vi "PH_IEEE1394Camera.PC Show Image.vi"(0 "i ref in":refnum<vi>, 2 "Show Image":bool, 5 "error IO":errorcluster) -> (14 "i ref out":refnum<vi>, 19 "error out":errorcluster)   [LabVIEW 2014]
doc: "This is the Proc Case \"Show Image\"."
uses:
  PH_IEEE1394Camera.lvlib
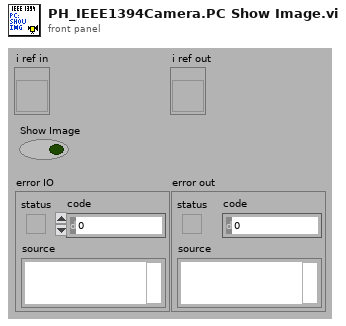
[diagram p1: front panel]
types:
  T1 = typedef "PH_IEEE1394Camera.lvlib/PH_IEEE1394Camera.i attribute.ctl" = cluster{"Gui Refs":cluster{"Cam name (Machinery)":refnum<vi>, "Start Cam":refnum<vi>, "Brightness":refnum<vi>, "Shutter":refnum<vi>, "Gain":refnum<vi>, "Center of Gravity":refnum<vi>, "Serial No":refnum<vi>, "Cam Name":refnum<vi>, "Connect":refnum<vi>, "Cam Attributes":refnum<vi>, "Supported Video Modes":refnum<vi>, "Cam Model":refnum<vi>, "Trigger Polarity":refnum<vi>, "Trigger Mode":refnum<vi>, "Trigger Timeout":refnum<vi>, "Bit Depth":refnum<vi>, "Video Mode":refnum<vi>, "Top":refnum<vi>, "Bottom":refnum<vi>, "Left":refnum<vi>, "Right":refnum<vi>, "Set ROI to Maximum":refnum<vi>}, "Cam":cluster{"Name (machinery)":string, "Serial Number":dbl, "IMAQ1394 Session":T2, "Restart":bool, "Supported Video Modes":cluster{"Video Mode":u32, "Video Mode Name":string}[], "Cam Model":string, "Readable Attributes":cluster{"Attribute Type":T3, "Attribute Name":string}[], "Writable Attributes":cluster{"Attribute Type":T3, "Attribute Name":string}[], "Read/Write Attributes":bool, "Attribute of Interest ":string, "Cam Attributes":cluster{"Video Mode":cluster{"Name":string, " Value":u32}, "Brightness":cluster{"Name":string, " Value":dbl}, "Gain":cluster{"Name":string, " Value":dbl}, "Shutter":cluster{"Name":string, " Value":dbl}, "Trigger Pol":cluster{"Name":string, " Value":u32}, "Trigger Mode":cluster{"Name":string, " Value":u32}, "Timeout":cluster{"Name":string, " Value":u32}, "Bit Depth":cluster{"Name":string, " Value":u32}, "Pixel Bits":cluster{"Name":string, " Value":bool}, "Pixel Bytes":cluster{"Name":string, " Value":bool}, "Left":cluster{"Name":string, " Value":u32, "Max":u32, "Min":u32}, "Right":cluster{"Name":string, " Value":u32, "Max":u32, "Min":u32}, "Top":cluster{"Name":string, " Value":u32, "Max":u32, "Min":u32}, "Bottom":cluster{"Name":string, " Value":u32, "Max":u32, "Min":u32}}}, "Refs Cam Attributes":cluster{"Selector":refnum<vi>, "Get / Set":refnum<vi>, "Set Num":refnum<vi>, "Set String / Command":refnum<vi>, "Set Bool":refnum<vi>, "Changed?":refnum<vi>, "Get: Read?":refnum<vi>, "Get Num":refnum<vi>, "Get Maximum":refnum<vi>, "Get Minimum":refnum<vi>, "EnumStrings":refnum<vi>, "EnumValues":refnum<vi>, "Get String / Command":refnum<vi>, "Get Bool":refnum<vi>, "Get Unit":refnum<vi>, "Get Description":refnum<vi>, "Cam Attributes Do it":refnum<vi>}}
  T2 = typedef "IMAQdx.ctl" = refnum<k21>
  T3 = typedef "NI_Vision_Acquisition_Software.lvlib/IMAQdx Attribute Type.ctl" = enum32{"U32", "I64", "DBL", "String", "Enum", "Bool", "Command"}
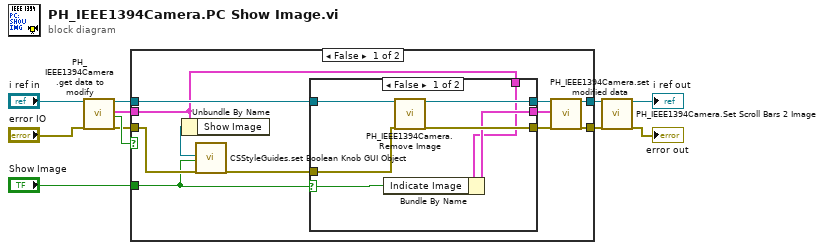
[diagram p0: block diagram]
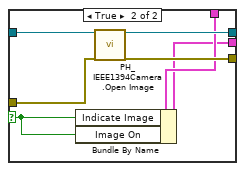
[diagram p2: hidden frame]
diagram:
  n1 = call "PH_IEEE1394Camera.get data to modify.vi"("i ref in"="i ref in", "error in (no error)"="error IO") -> ("i ref out"=w4:refnum<vi>, "i attribute"=w5:T1, "timed out"=w7:bool, "error out"=w3:errorcluster)  [unwired: 14 in]
  n2 = case shown="False" w7 {
    tunnel: w3 -> [w19 w37]
    tunnel: [w22 w37] -> w11
    tunnel: w4 -> [w18 w38]
    tunnel: [w21 w38] -> w9
    tunnel: w5 -> [w12 _]
    tunnel: "Show Image" -> [w16 _]
    frame False {
      n3 = Unbundle By Name(w12) -> ("Show Image"=w20:refnum<vi>)
      n4 = call "CSStyleGuides.set Boolean Knob GUI Object.vi"("Boolean Knob GUI Ref"=w20, "Value"=w16, "error in (no error)"=w19) -> ("error out"=w15:errorcluster)  [unwired: 16 in]
      n5 = case shown="False" w16 {
        selector: w16 -> [w25 w30]
        tunnel: w15 -> [w29 w33]
        tunnel: [w28 w36] -> w14
        tunnel: w18 -> [w27 w35]
        tunnel: [w26 w34] -> w17
        tunnel: [w24 w31] -> w13
        tunnel: w12 -> [w23 w32]
        frame False {
          n6 = Bundle By Name(cluster=w23, "Indicate Image"=w25) -> (w24:T1)
          n7 = call "PH_IEEE1394Camera.Remove Image.vi"("i ref in"=w27, "error in"=w29) -> ("i ref out"=w26:refnum<vi>, "error out"=w28:errorcluster)  [unwired: 16 in]
        }
        frame True {
          n8 = Bundle By Name(cluster=w32, "Indicate Image"=w30, "Image On"=w30) -> (w31:T1)
          n9 = call "PH_IEEE1394Camera.Open Image.vi"("i ref in"=w35, "error in"=w33) -> ("i ref out"=w34:refnum<vi>, "error out"=w36:errorcluster)  [unwired: 16 in]
        }
      }
      n10 = call "PH_IEEE1394Camera.set modified data.vi"("i ref in"=w17, "i attribute"=w13, "error in (no error)"=w14) -> ("i ref out"=w21:refnum<vi>, "error out"=w22:errorcluster)  [unwired: 15 in]
    }
    frame True {
    }
  }
  n11 = call "PH_IEEE1394Camera.Set Scroll Bars 2 Image.vi"("i ref in"=w9, "error in (no error)"=w11) -> ("i ref out"=→"i ref out":refnum<vi>, "error out"=→"error out":errorcluster)  [unwired: 16 in]
